vi "subWriteErrorMessage.vi"(8 "error in (no error)":errorcluster, 9 "Restricted Object":string, 10 "VI Name":string, 11 "CLI in":refnum<class "CLI.lvclass">) -> (0 "error out":errorcluster, 3 "CLI out":refnum<class "CLI.lvclass">)   [LabVIEW 2014, in "lvbuildsecurity.lvlib"]
uses:
  lvbuildsecurity.lvlib
  <vilib>/Wiresmith Technology/LabVIEW CLI/CLI Class/CLI.lvclass
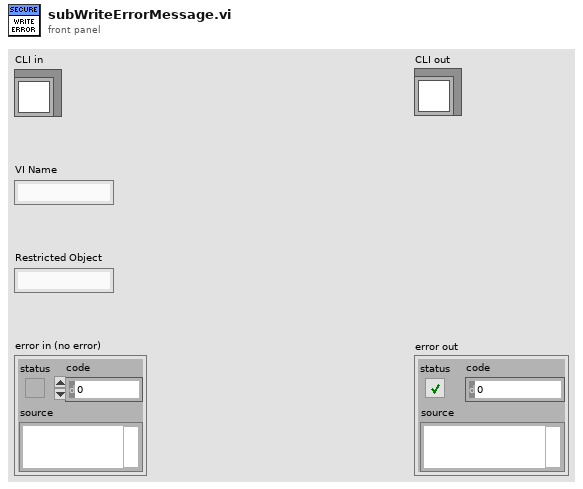
[diagram p1: front panel]
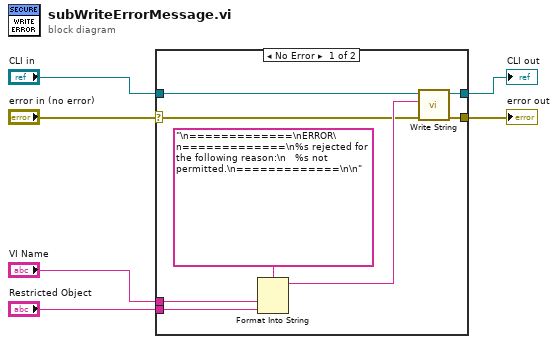
[diagram p0: block diagram]
diagram:
  n1 = case shown="No Error" "error in (no error)" {
    selector: "error in (no error)" -> [w7 w15]
    tunnel: "CLI in" -> [w12 w16]
    tunnel: "VI Name" -> [w11 _]
    tunnel: "Restricted Object" -> [w10 _]
    tunnel: [w9 w15] -> w1
    tunnel: [w8 w16] -> w2
    frame No Error {
      n2 = Format Into String(format string="\n=============\nERROR\n=============\n%s rejected for the following reason:\n   %s not permitted.\n=============\n\n", w11, w10) -> (resulting string=w13:string)  [unwired: 2 in, 1 out]
      n3 = call <vilib>:"Write String.vi"("error in (no error)"=w7, "Text to Write"=w13, "CLI in"=w12) -> ("error out"=w9:errorcluster, "CLI out"=w8:refnum<class "CLI.lvclass">)  [unwired: 7 in]
    }
    frame Error {
    }
  }
  "CLI out" <- w2
  "error out" <- w1
